vi "rt_main.vi"() -> ()   [LabVIEW 2013]
uses:
  <vilib>/dex/Flush And Wait Empty Condition.ctl
  <vilib>/Platform/TimedLoop/XDataNode/timing_clust.ctl
  <vilib>/Platform/TimedLoop/XDataNode/nitl_modes.ctl
  <vilib>/Platform/TimedLoop/XDataNode/wakeup.ctl
  <vilib>/FPGAPlugInAG/sbRIO-9636/niLvFpga_Open_sbRIO-9636.vi
  <vilib>/rvi/interface/common/dynamic/niFpgaDynamicAddResources.vi
  <vilib>/rvi/interface/common/niFpgaWaitOnOcc.vi
  <vilib>/Utility/error.llb/Error Cluster From Error Code.vi
  <vilib>/rvi/errors/niLvFpgaAdjustHostInterfaceError.vi
  <vilib>/FPGAPlugInAG/Dynamic/niLvFpga_Close_Dynamic.vi
  <vilib>/Platform/TimedLoop/XDataNode/XDataNode.xnode
  <vilib>/rvi/interface/nirviOpenFPGA/nirviOpenFPGA.xnode
  FPGA Bitfiles/ControlPanelproj_FPGATarget_fpgamain_xa8pjD6vMWE.lvbitx
  fpga_main.vi
  <vilib>/rvi/interface/nirviMethod/nirviMethod.xnode
  <vilib>/rvi/interface/nirviReadWriteControl/nirviReadWriteControl.xnode
  <vilib>/rvi/interface/nirviCloseFPGA/nirviCloseFPGA.xnode
  <vilib>/Platform/TimedLoop/XDataNode/XDNodeRunTimeDep.lvlib
  <vilib>/rvi/errors/niLvFpgaMergeErrorWithErrorCode.vi
  <vilib>/FPGAPlugInAG/Dynamic/niLvFpga_ReadFifo_Dynamic.vi
  <vilib>/FPGAPlugInAG/Dynamic/niLvFpga_ConfigureFifo_Dynamic.vi
  NiFpgaLv.dll
  <vilib>/rvi/interface/Simulation/niFpgaSimulationCallBeginRW.vi
  <vilib>/FPGAPlugInAG/Dynamic/niLvFpga_WriteFifo_Dynamic.vi
panel:
  in  "Ignore Minutes and Seconds":bool
  in  "HrStartDispense":i64
  in  "HrGetOrigDispense":i64
  in  "Ignore Minutes and Seconds for ContUpdate":bool
  in  "HrToUpdateCont":i64
  out "Time in 64 Bits":i64
  out "Skip Count":i32
  out "Elements Remaining":u32
  out "Number of Elements":u32
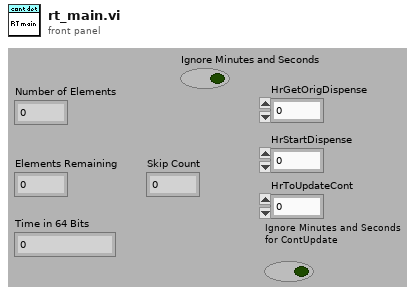
[diagram p1: front panel]
types:
  T1 = typedef "Flush And Wait Empty Condition.ctl" = u8
  T2 = typedef "XDNodeRunTimeDep.lvlib/timing_clust.ctl" = cluster{"Expected End [f-1]":u64, "Actual End [f-1]":u64, "Finished Late? [f-1]":bool, "Expected End [i-1]":u64, "Actual End [i-1]":u64, "Finished Late? [i-1]":bool, "Expected Start [i]":u64, "Actual Start [i]":u64, "Expected Start [f]":u64, "Actual Start [f]":u64, "Source Name":string, "Structure Name":string, "Period":i64, "Deadline":i64, "Offset":i64, "Start":i64, "Priority":i32, "Timeout":i32, "Mode":T3, "Wakeup Reason":T4, "Error":errorcluster, "Source Type":string, "Secondary Source Type":string, "Global End Time":u64, "Global Start Time":u64, "Frame Duration":u64, "Iteration Duration":u64, "Assigned CPU":i32, "I/O Scan Engine Mode":u32}
  T3 = typedef "XDNodeRunTimeDep.lvlib/nitl_modes.ctl" = enum32{"No Change", "Process missed periods, maintain original phase", "Discard missed periods, maintain original phase", "Process missed periods, ignore original phase", "Discard missed periods, ignore original phase"}
  T4 = typedef "XDNodeRunTimeDep.lvlib/wakeup.ctl" = enum32{"Normal", "Aborted", "Asynchronous wakeup", "Timing source error", "Timed loop error", "Timeout"}
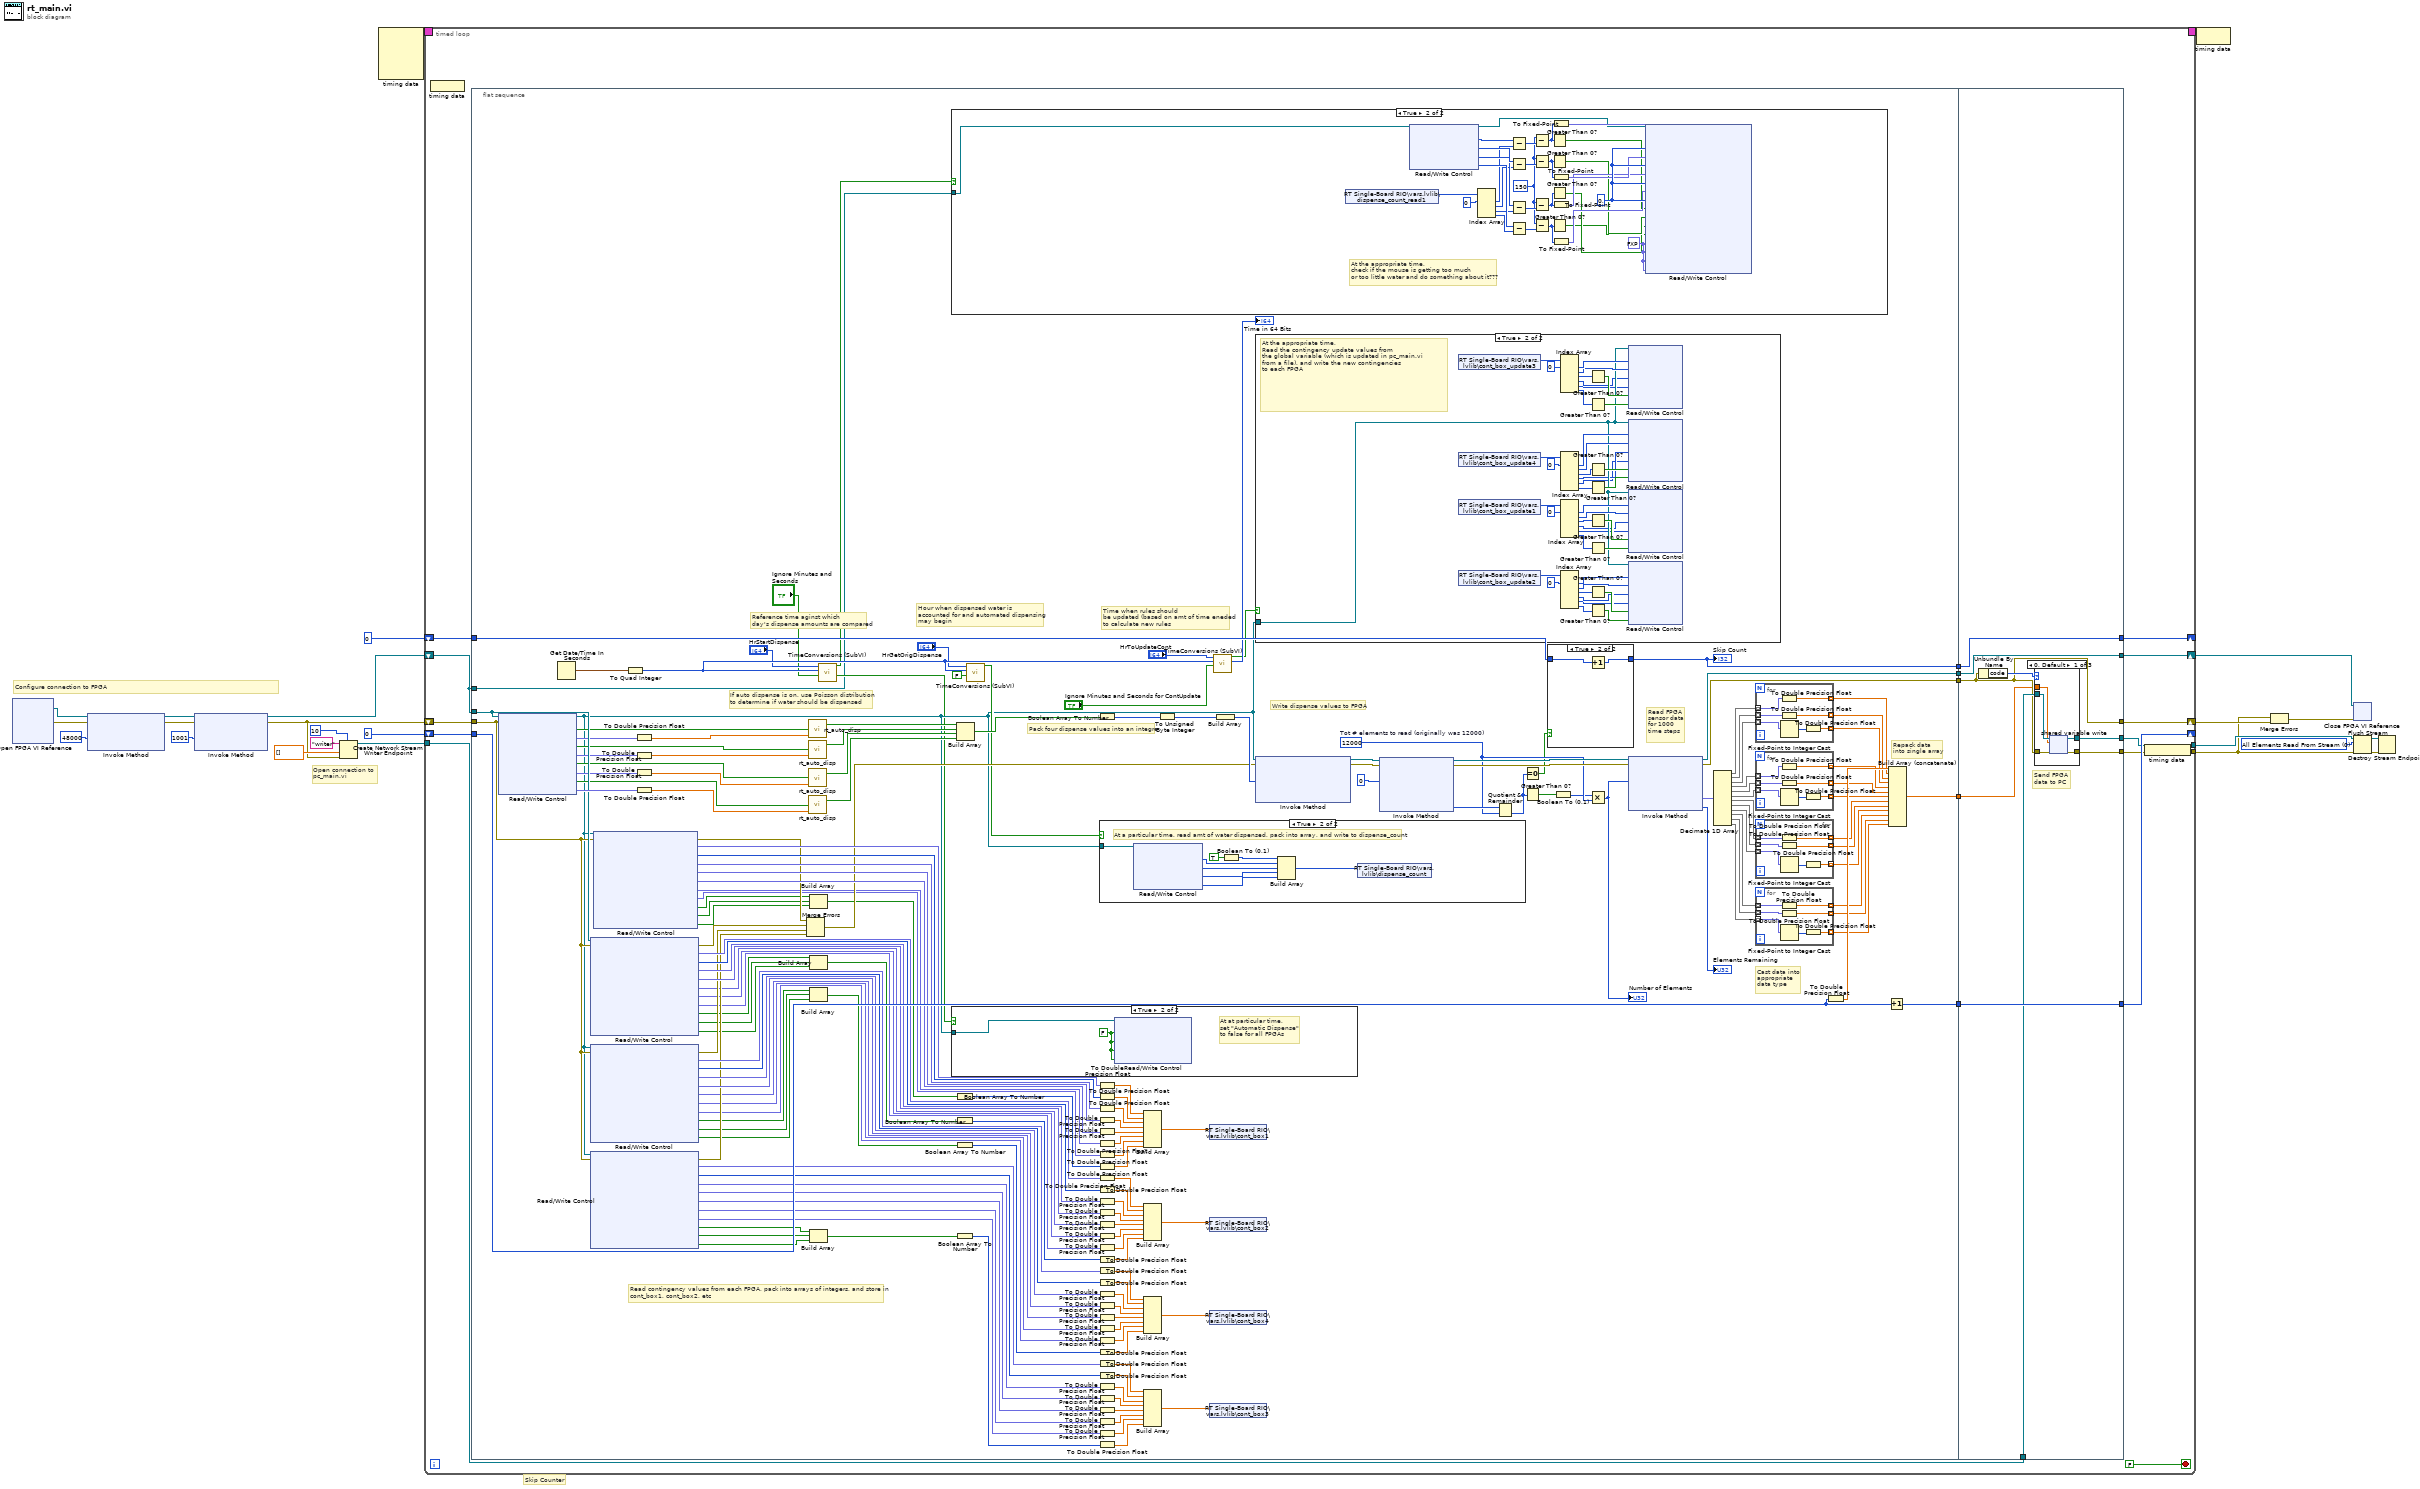
[diagram p0: block diagram]
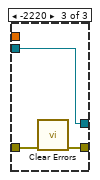
[diagram p8: hidden frame]
diagram:
  w5 = T1 0 items=["All Elements Read From Stream", "All Elements Available for Reading"] ("wait condition")
  # "Open connection to \npc_main.vi"
  # "Configure connection to FPGA"
  # "Skip Counter"
  n1 = xnode "Open FPGA VI Reference"() -> ("FPGA VI Reference Out"=w15:refnum<k20>, "error out"=w14:errorcluster)  [unwired: 2 in]
  n2 = xnode "Invoke Method"("FPGA VI Reference In"=w15, "error in"=w14, "Requested Depth"=u32 48000) -> ("FPGA VI Reference Out"=w9:refnum<k20>, "error out"=w10:errorcluster)  [unwired: 1 out]
  n3 = xnode "Invoke Method"("FPGA VI Reference In"=w9, "error in"=w10, "Requested Depth"=u32 1001) -> ("FPGA VI Reference Out"=w8:refnum<k20>, "error out"=w7:errorcluster)  [unwired: 1 out]
  n4 = Create Network Stream Writer Endpoint(7:10 ("writer buffer size"), 8:w7, 9:dbl[] [], 11:"writer" ("writer name")) -> (3:w6:refnum<k21>)  [unwired: 3 in, 1 out]
  n5 = node-c288() -> (w24:T2)  [unwired: 4 in]
  n6 = timed-loop {
    shift-right: [w41] -> w18
    shift-left: w7 -> [w35]
    timing: w24 -> [_]
    timing-out: [_] -> w23
    shift-right: [w40] -> w22
    shift-left: w8 -> [w25]
    shift-right: [w39] -> _
    shift-left: u32 0 ("index") -> [w38]
    shift-right: [w36] -> _
    shift-left: 0 -> [w37]
    tunnel: w6 -> [w30]
    tunnel: [w29] -> w1
    tunnel: [w28] -> w2
    stop <- FALSE stop-if-true
    n7 = node-c288() -> ()  [unwired: 1 in]
    n8 = flat-sequence {
      tunnel: w38 -> [w205]
      tunnel: w37 -> [w198]
      tunnel: w25 -> [w164]
      tunnel: w35 -> [w120]
      tunnel: [w50] -> w34
      tunnel: [w206] -> w33
      tunnel: [w196] -> w32
      tunnel: [w95] -> w27
      tunnel: [w94] -> w26
      tunnel: w25 -> [w44]
      tunnel: [w333] -> w36
      tunnel: [w334] -> w39
      tunnel: [w335] -> w40
      tunnel: [w328] -> w41
      tunnel: w34 -> [w335]
      tunnel: w33 -> [w334]
      tunnel: w32 -> [w333]
      tunnel: w30 -> [w331]
      tunnel: [w330] -> w29
      tunnel: [w329] -> w28
      tunnel: w27 -> [w328]
      tunnel: w26 -> [w327]
      frame #0 {
        w199 = u32 12000  # Tot # elements to read (originally was 12000)
        # "Reference time aginst which\nday's dispense amounts are compared"
        # "Hour when dispensed water is \naccounted for and automated dispensing\nmay begin"
        # "Time when rules should\nbe updated (based on amt of time eneded\nto calculate new rules"
        # "Read contingency values from each FPGA, pack into arrays of integers, and store in\ncont_box1, cont_box2, etc"
        # "Repack data\ninto single array"
        # "Cast data into\nappropriate\ndata type"
        # "Read FPGA \nsensor data\nfor 1000 \ntime steps"
        # "Write dispense values to FPGA"
        # "Pack four dispense values into an integre"
        # "If auto dispense is on, use Poisson distribution\nto determine if water should be dispensed"
        n9 = xnode "Read/Write Control"("FPGA VI Reference In"=w164, "error in"=w120) -> ("FPGA VI Reference Out"=w49:refnum<k20>, "Automatic Dispense 1"=w111:bool, "Mean 1"=w112:fxp<+,22,9>, "Automatic Dispense 2"=w110:bool, "Mean 2"=w109:fxp<+,22,9>, "Automatic Dispense 3"=w108:bool, "Mean 3"=w107:fxp<+,22,9>, "Automatic Dispense 4"=w113:bool, "Mean 4"=w180:fxp<+,22,9>)  [unwired: 1 out]
        n10 = Get Date/Time In Seconds() -> (seconds since 1Jan1904=w57:timestamp)
        n11 = xnode "Read/Write Control"("FPGA VI Reference In"=w164, "error in"=w120) -> ("error out"=w118:errorcluster, "Outer Threshold 2"=w163:fxp<+,22,9>, "Hold Duration 2"=w161:i16, "Inner Threshold 2"=w159:fxp<+,22,9>, "Min Angle 2"=w156:fxp<+,9,9>, "Max Angle 2"=w60:fxp<+,9,9>, "Min Angle 2 2"=w59:fxp<+,9,9>, "Max Angle 2 2"=w58:fxp<+,9,9>, "Sequence Override 2"=w104:bool, "Override Fail when moved out 2"=w103:bool, "Override Approach 2"=w76:bool)  [unwired: 1 out]
        n12 = xnode "Read/Write Control"("FPGA VI Reference In"=w49, "error in"=w120) -> ("error out"=w119:errorcluster, "Outer Threshold 4"=w132:fxp<+,22,9>, "Hold Duration 4"=w130:i16, "Inner Threshold 4"=w128:fxp<+,22,9>, "Min Angle 4"=w125:fxp<+,9,9>, "Max Angle 4"=w63:fxp<+,9,9>, "Min Angle 4 2"=w62:fxp<+,9,9>, "Max Angle 4 2"=w61:fxp<+,9,9>, "Sequence Override 4"=w96:bool, "Override Fail when moved out 4"=w80:bool, "Override Approach 4"=w79:bool)  [unwired: 1 out]
        n13 = xnode "Read/Write Control"("FPGA VI Reference In"=w49, "error in"=w120) -> ("error out"=w121:errorcluster, "Outer Threshold 3"=w142:fxp<+,22,9>, "Hold Duration 3"=w140:i16, "Inner Threshold 3"=w138:fxp<+,22,9>, "Min Angle 3"=w135:fxp<+,9,9>, "Max Angle 3"=w66:fxp<+,9,9>, "Min Angle 3 2"=w65:fxp<+,9,9>, "Max Angle 3 2"=w64:fxp<+,9,9>, "Sequence Override 3"=w100:bool, "Override Fail when moved out 3"=w99:bool, "Override Approach 3"=w77:bool)  [unwired: 1 out]
        n14 = xnode "Read/Write Control"("FPGA VI Reference In"=w49, "error in"=w120) -> ("error out"=w117:errorcluster, "Outer Threshold 1"=w153:fxp<+,22,9>, "Hold Duration 1"=w151:i16, "Inner Threshold 1"=w149:fxp<+,22,9>, "Min Angle 1"=w146:fxp<+,9,9>, "Max Angle 1"=w145:fxp<+,9,9>, "Min Angle 1 2"=w82:fxp<+,9,9>, "Max Angle 1 2"=w83:fxp<+,9,9>, "Sequence Override 1"=w116:bool, "Override Fail when moved out"=w78:bool, "Override Approach 1"=w81:bool)  [unwired: 1 out]
        n15 = To Quad Integer(1:w57) -> (0:w53:i64)
        n16 = To Double Precision Float(number=w112) -> (double precision float=w179:dbl)
        n17 = To Double Precision Float(number=w109) -> (double precision float=w187:dbl)
        n18 = To Double Precision Float(number=w107) -> (double precision float=w186:dbl)
        n19 = To Double Precision Float(number=w180) -> (double precision float=w181:dbl)
        n20 = Merge Errors(w117, w118, w119, w121) -> (w122:errorcluster)
        n21 = call "rt_auto_disp.vi"("Mean"=w179, "Enable"=w111) -> ("Dispense"=w178:bool)  [unwired: 2 in]
        n22 = call "rt_auto_disp.vi"("Mean"=w187, "Enable"=w110) -> ("Dispense"=w184:bool)  [unwired: 2 in]
        n23 = call "rt_auto_disp.vi"("Mean"=w186, "Enable"=w108) -> ("Dispense"=w185:bool)  [unwired: 2 in]
        n24 = call "rt_auto_disp.vi"("Mean"=w181, "Enable"=w113) -> ("Dispense"=w177:bool)  [unwired: 2 in]
        n25 = Build Array(w116, w78, w81) -> (w115:bool[])
        n26 = Build Array(w104, w103, w76) -> (w106:bool[])
        n27 = Build Array(w96, w80, w79) -> (w98:bool[])
        n28 = Build Array(w100, w99, w77) -> (w102:bool[])
        n29 = call "TimeConversions (SubVI).vi"("Ignore Minutes and Seconds"="Ignore Minutes and Seconds", "Current time"=w53, "HrToUpdate"="HrStartDispense") -> ("Delay_cont"=w47:bool, "Boolean"=w48:bool)  [unwired: 6 in, 1 out]
        n30 = case shown="True" w48 {
          tunnel: w44 -> [_ w219]
          frame False {
          }
          frame True {
            w221 = u16 150 ("x")
            w234 = fxp<+,22,9> 10.0 ("Mean 4")
            w235 = i16 0 ("Automated Pellets Dispensed 2")
            # "At the appropriate time,\ncheck if the mouse is getting too much \nor too little water and do something about it???"
            n31 = shared-variable "RT Single-Board RIO\\vars.lvlib\\dispense_count_read1"() -> (w220:u16[])  [unwired: 1 in, 1 out]
            n32 = xnode "Read/Write Control"("FPGA VI Reference In"=w219) -> ("FPGA VI Reference Out"=w218:refnum<k20>, "Pellets Dispensed 1"=w244:u16, "Pellets Dispensed 2"=w243:u16, "Pellets Dispensed 3"=w242:u16, "Pellets Dispensed 4"=w241:u16)  [unwired: 1 in, 1 out]
            n33 = Index Array(array=w220, index #1=0 ("index")) -> (element #1=w239:u16, element #2=w238:u16, element #3=w237:u16, element #4=w236:u16)  [unwired: 3 in]
            n34 = Subtract(x=w244, y=w239) -> (x-y=w222:u16)
            n35 = Subtract(x=w243, y=w238) -> (x-y=w223:u16)
            n36 = Subtract(x=w242, y=w237) -> (x-y=w224:u16)
            n37 = Subtract(x=w241, y=w236) -> (x-y=w225:u16)
            n38 = Subtract(x=w221, y=w222) -> (x-y=w214:i16)
            n39 = Subtract(x=w221, y=w223) -> (x-y=w215:i16)
            n40 = Subtract(x=w221, y=w224) -> (x-y=w217:i16)
            n41 = Subtract(x=w221, y=w225) -> (x-y=w216:i16)
            n42 = Greater Than 0?(x=w214) -> (x > 0?=w229:bool)
            n43 = Greater Than 0?(x=w215) -> (x > 0?=w228:bool)
            n44 = Greater Than 0?(x=w217) -> (x > 0?=w227:bool)
            n45 = Greater Than 0?(x=w216) -> (x > 0?=w226:bool)
            n46 = To Fixed-Point(number=w214) -> (fixed-point=w233:fxp<+,10,10>)  [unwired: 1 in]
            n47 = To Fixed-Point(number=w215) -> (fixed-point=w232:fxp<+,10,10>)  [unwired: 1 in]
            n48 = To Fixed-Point(number=w217) -> (fixed-point=w231:fxp<+,10,10>)  [unwired: 1 in]
            n49 = To Fixed-Point(number=w216) -> (fixed-point=w230:fxp<+,10,10>)  [unwired: 1 in]
            n50 = xnode "Read/Write Control"("FPGA VI Reference In"=w218, "Automated Pellets Target 1"=w233, "Automated Pellets Dispensed 1"=w235, "Automated Pellets Target 2"=w232, "Automated Pellets Dispensed 2"=w235, "Automated Pellets Target 3"=w231, "Automated Pellets Dispensed 3"=w235, "Automated Pellets Target 4"=w230, "Automated Pellets Dispensed 4"=w235, "Automatic Dispense 1"=w229, "Automatic Dispense 2"=w228, "Automatic Dispense 3"=w227, "Automatic Dispense 4"=w226, "Mean 1"=w234, "Mean 2"=w234, "Mean 3"=w234, "Mean 4"=w234) -> ()  [unwired: 1 in, 2 out]
          }
        }
        n51 = case shown="True" w47 {
          tunnel: w49 -> [_ w253]
          frame False {
          }
          frame True {
            w254 = FALSE ("Automatic Dispense 1")
            # "At at particular time,\nset \"Automatic Dispense\"\nto false for all FPGAs"
            n52 = xnode "Read/Write Control"("FPGA VI Reference In"=w253, "Automatic Dispense 1"=w254, "Automatic Dispense 2"=w254, "Automatic Dispense 3"=w254, "Automatic Dispense 4"=w254) -> ()  [unwired: 1 in, 2 out]
          }
        }
        n53 = Boolean Array To Number(Boolean array=w115) -> (number=w114:u32)
        n54 = Boolean Array To Number(Boolean array=w106) -> (number=w105:u32)
        n55 = Boolean Array To Number(Boolean array=w98) -> (number=w97:u32)
        n56 = Boolean Array To Number(Boolean array=w102) -> (number=w101:u32)
        n57 = Build Array(w178, w184, w185, w177) -> (w188:bool[])
        n58 = call "TimeConversions (SubVI).vi"("Ignore Minutes and Seconds"=FALSE, "Current time"=w53, "HrToUpdate"="HrGetOrigDispense") -> ("Boolean"=w51:bool)  [unwired: 6 in, 2 out]
        n59 = Boolean Array To Number(Boolean array=w188) -> (number=w189:u32)
        n60 = To Double Precision Float(number=w153) -> (double precision float=w152:dbl)
        n61 = To Double Precision Float(number=w151) -> (double precision float=w150:dbl)
        n62 = To Double Precision Float(number=w149) -> (double precision float=w148:dbl)
        n63 = To Double Precision Float(number=w146) -> (double precision float=w147:dbl)
        n64 = To Double Precision Float(number=w145) -> (double precision float=w144:dbl)
        n65 = To Double Precision Float(number=w82) -> (double precision float=w84:dbl)
        n66 = To Double Precision Float(number=w83) -> (double precision float=w85:dbl)
        n67 = To Double Precision Float(number=w114) -> (double precision float=w86:dbl)
        n68 = To Double Precision Float(number=w163) -> (double precision float=w162:dbl)
        n69 = To Double Precision Float(number=w161) -> (double precision float=w160:dbl)
        n70 = To Double Precision Float(number=w159) -> (double precision float=w158:dbl)
        n71 = To Double Precision Float(number=w156) -> (double precision float=w157:dbl)
        n72 = To Double Precision Float(number=w60) -> (double precision float=w155:dbl)
        n73 = To Double Precision Float(number=w59) -> (double precision float=w73:dbl)
        n74 = To Double Precision Float(number=w58) -> (double precision float=w74:dbl)
        n75 = To Double Precision Float(number=w105) -> (double precision float=w75:dbl)
        n76 = To Double Precision Float(number=w132) -> (double precision float=w131:dbl)
        n77 = To Double Precision Float(number=w130) -> (double precision float=w129:dbl)
        n78 = To Double Precision Float(number=w128) -> (double precision float=w127:dbl)
        n79 = To Double Precision Float(number=w125) -> (double precision float=w126:dbl)
        n80 = To Double Precision Float(number=w63) -> (double precision float=w124:dbl)
        n81 = To Double Precision Float(number=w62) -> (double precision float=w71:dbl)
        n82 = To Double Precision Float(number=w61) -> (double precision float=w70:dbl)
        n83 = To Double Precision Float(number=w97) -> (double precision float=w72:dbl)
        n84 = To Double Precision Float(number=w142) -> (double precision float=w141:dbl)
        n85 = To Double Precision Float(number=w140) -> (double precision float=w139:dbl)
        n86 = To Double Precision Float(number=w138) -> (double precision float=w137:dbl)
        n87 = To Double Precision Float(number=w135) -> (double precision float=w136:dbl)
        n88 = To Double Precision Float(number=w66) -> (double precision float=w134:dbl)
        n89 = To Double Precision Float(number=w65) -> (double precision float=w67:dbl)
        n90 = To Double Precision Float(number=w64) -> (double precision float=w68:dbl)
        n91 = To Double Precision Float(number=w101) -> (double precision float=w69:dbl)
        n92 = case shown="True" w51 {
          tunnel: w49 -> [_ w252]
          frame False {
          }
          frame True {
            # "At a particular time, read amt of water dispensed, pack into array, and write to dispense_count"
            n93 = xnode "Read/Write Control"("FPGA VI Reference In"=w252) -> ("Pellets Dispensed 1"=w248:u16, "Pellets Dispensed 2"=w249:u16, "Pellets Dispensed 3"=w250:u16, "Pellets Dispensed 4"=w251:u16)  [unwired: 1 in, 2 out]
            n94 = Boolean To (0,1)(Boolean=TRUE) -> (0, 1=w246:i16)
            n95 = Build Array(w246, w248, w249, w250, w251) -> (w245:u16[])
            n96 = shared-variable "RT Single-Board RIO\\vars.lvlib\\dispense_count"(w245) -> ()  [unwired: 1 in, 1 out]
          }
        }
        n97 = Build Array(w152, w150, w148, w147, w144, w84, w85, w86) -> (w143:dbl[])
        n98 = Build Array(w162, w160, w158, w157, w155, w73, w74, w75) -> (w154:dbl[])
        n99 = Build Array(w131, w129, w127, w126, w124, w71, w70, w72) -> (w123:dbl[])
        n100 = Build Array(w141, w139, w137, w136, w134, w67, w68, w69) -> (w133:dbl[])
        n101 = To Unsigned Byte Integer(number=w189) -> (unsigned 8bit integer=w183:u8)
        n102 = shared-variable "RT Single-Board RIO\\vars.lvlib\\cont_box1"(w143) -> ()  [unwired: 1 in, 1 out]
        n103 = shared-variable "RT Single-Board RIO\\vars.lvlib\\cont_box2"(w154) -> ()  [unwired: 1 in, 1 out]
        n104 = shared-variable "RT Single-Board RIO\\vars.lvlib\\cont_box4"(w123) -> ()  [unwired: 1 in, 1 out]
        n105 = shared-variable "RT Single-Board RIO\\vars.lvlib\\cont_box3"(w133) -> ()  [unwired: 1 in, 1 out]
        n106 = call "TimeConversions (SubVI).vi"("Ignore Minutes and Seconds"="Ignore Minutes and Seconds for ContUpdate", "Current time"=w53, "HrToUpdate"="HrToUpdateCont") -> ("Time in 64 Bits"=→"Time in 64 Bits":i64, "Boolean"=w46:bool)  [unwired: 6 in, 1 out]
        n107 = Build Array(w183) -> (w182:u8[])
        n108 = case shown="True" w46 {
          tunnel: w49 -> [_ w271]
          frame False {
          }
          frame True {
            # "At the appropriate time,\nRead the contingency update values from\nthe global variable (which is updated in pc_main.vi\nfrom a file), and write the new contingencies\nto each FPGA"
            n109 = shared-variable "RT Single-Board RIO\\vars.lvlib\\cont_box_update3"() -> (w273:i32[])  [unwired: 1 in, 1 out]
            n110 = shared-variable "RT Single-Board RIO\\vars.lvlib\\cont_box_update4"() -> (w272:i32[])  [unwired: 1 in, 1 out]
            n111 = shared-variable "RT Single-Board RIO\\vars.lvlib\\cont_box_update1"() -> (w275:i32[])  [unwired: 1 in, 1 out]
            n112 = shared-variable "RT Single-Board RIO\\vars.lvlib\\cont_box_update2"() -> (w274:i32[])  [unwired: 1 in, 1 out]
            n113 = Index Array(array=w273, index #1=0 ("index")) -> (element #1=w279:i32, element #2=w278:i32, element #3=w262:i32, element #4=w260:i32, element #5=w259:i32, element #6=w261:i32)  [unwired: 5 in]
            n114 = Index Array(array=w272, index #1=0 ("index")) -> (element #1=w281:i32, element #2=w280:i32, element #3=w270:i32, element #4=w269:i32, element #5=w268:i32, element #6=w267:i32)  [unwired: 5 in]
            n115 = Index Array(array=w275, index #1=0 ("index")) -> (element #1=w283:i32, element #2=w282:i32, element #3=w266:i32, element #4=w264:i32, element #5=w263:i32, element #6=w265:i32)  [unwired: 5 in]
            n116 = Index Array(array=w274, index #1=0 ("index")) -> (element #1=w276:i32, element #2=w277:i32, element #3=w258:i32, element #4=w256:i32, element #5=w255:i32, element #6=w257:i32)  [unwired: 5 in]
            n117 = Greater Than 0?(x=w262) -> (x > 0?=w292:bool)
            n118 = Greater Than 0?(x=w261) -> (x > 0?=w293:bool)
            n119 = Greater Than 0?(x=w270) -> (x > 0?=w295:bool)
            n120 = Greater Than 0?(x=w267) -> (x > 0?=w294:bool)
            n121 = Greater Than 0?(x=w266) -> (x > 0?=w289:bool)
            n122 = Greater Than 0?(x=w265) -> (x > 0?=w288:bool)
            n123 = Greater Than 0?(x=w258) -> (x > 0?=w291:bool)
            n124 = Greater Than 0?(x=w257) -> (x > 0?=w290:bool)
            n125 = xnode "Read/Write Control"("FPGA VI Reference In"=w271, "Min Angle 3"=w279, "Max Angle 3"=w278, "Min Angle 3 2"=w260, "Max Angle 3 2"=w259, "CCW(T)  3"=w292, "CCW(T)  3 2"=w293) -> ()  [unwired: 1 in, 2 out]
            n126 = xnode "Read/Write Control"("FPGA VI Reference In"=w271, "Min Angle 4"=w281, "Max Angle 4"=w280, "Min Angle 4 2"=w269, "Max Angle 4 2"=w268, "CCW(T)  4"=w295, "CCW(T)  4 2"=w294) -> ()  [unwired: 1 in, 2 out]
            n127 = xnode "Read/Write Control"("FPGA VI Reference In"=w271, "Min Angle 1"=w283, "Max Angle 1"=w282, "Min Angle 1 2"=w264, "Max Angle 1 2"=w263, "CCW(T) 1"=w289, "CCW(T) 1 2"=w288) -> ()  [unwired: 1 in, 2 out]
            n128 = xnode "Read/Write Control"("FPGA VI Reference In"=w271, "Min Angle 2"=w276, "Max Angle 2"=w277, "Min Angle 2 2"=w256, "Max Angle 2 2"=w255, "CCW(T)  2"=w291, "CCW(T)  2 2"=w290) -> ()  [unwired: 1 in, 2 out]
          }
        }
        n129 = xnode "Invoke Method"("FPGA VI Reference In"=w49, "error in"=w122, "Data"=w182) -> ("FPGA VI Reference Out"=w208:refnum<k20>, "error out"=w207:errorcluster)  [unwired: 1 in, 1 out]
        n130 = xnode "Invoke Method"("FPGA VI Reference In"=w208, "error in"=w207, "Number of Elements"=u32 0) -> ("FPGA VI Reference Out"=w211:refnum<k20>, "error out"=w210:errorcluster, "Elements Remaining"=w212:u32)  [unwired: 1 in, 1 out]
        n131 = Quotient & Remainder(x=w212, y=w199) -> (floor(x/y)=w93:u32)  [unwired: 1 out]
        n132 = Equal To 0?(x=w93) -> (x = 0?=w197:bool)
        n133 = Greater Than 0?(x=w93) -> (x > 0?=w91:bool)
        n134 = case shown="True" w197 {
          tunnel: w198 -> [w310 w312]
          tunnel: [w310 w311] -> w196
          frame False {
          }
          frame True {
            n135 = Increment(x=w312) -> (x+1=w311:i32)
          }
        }
        "Skip Count" <- w196
        n136 = Boolean To (0,1)(Boolean=w91) -> (0, 1=w92:i16)
        n137 = Multiply(x=w92, y=w199) -> (x*y=w204:u32)
        "Number of Elements" <- w204
        n138 = xnode "Invoke Method"("FPGA VI Reference In"=w211, "error in"=w210, "Number of Elements"=w204) -> ("FPGA VI Reference Out"=w50:refnum<k20>, "error out"=w95:errorcluster, "Data"=w209:fxp<+/-,22,10>[], "Elements Remaining"=→"Elements Remaining":u32)  [unwired: 1 in]
        n139 = Decimate 1D Array(w209) -> (w89:fxp<+/-,22,10>[], w88:fxp<+/-,22,10>[], w87:fxp<+/-,22,10>[], w203:fxp<+/-,22,10>[], w202:fxp<+/-,22,10>[], w201:fxp<+/-,22,10>[], w176:fxp<+/-,22,10>[], w175:fxp<+/-,22,10>[], w174:fxp<+/-,22,10>[], w173:fxp<+/-,22,10>[], w172:fxp<+/-,22,10>[], w171:fxp<+/-,22,10>[])
        n140 = for {
          tunnel: w89 -> [w326] mode=indexing
          tunnel: w88 -> [w325] mode=indexing
          tunnel: w87 -> [w324] mode=indexing
          tunnel: [w321] -> w195 mode=indexing
          tunnel: [w320] -> w194 mode=indexing
          tunnel: [w322] -> w193 mode=indexing
          n141 = To Double Precision Float(number=w326) -> (double precision float=w321:dbl)
          n142 = To Double Precision Float(number=w325) -> (double precision float=w320:dbl)
          n143 = Fixed-Point to Integer Cast(1:w324) -> (0:w323:i32)
          n144 = To Double Precision Float(number=w323) -> (double precision float=w322:dbl)
        }
        n145 = for {
          tunnel: w203 -> [w319] mode=indexing
          tunnel: w202 -> [w318] mode=indexing
          tunnel: w201 -> [w317] mode=indexing
          tunnel: [w314] -> w192 mode=indexing
          tunnel: [w313] -> w191 mode=indexing
          tunnel: [w315] -> w190 mode=indexing
          n146 = To Double Precision Float(number=w319) -> (double precision float=w314:dbl)
          n147 = To Double Precision Float(number=w318) -> (double precision float=w313:dbl)
          n148 = Fixed-Point to Integer Cast(1:w317) -> (0:w316:i32)
          n149 = To Double Precision Float(number=w316) -> (double precision float=w315:dbl)
        }
        n150 = for {
          tunnel: w176 -> [w309] mode=indexing
          tunnel: w175 -> [w308] mode=indexing
          tunnel: w174 -> [w307] mode=indexing
          tunnel: [w304] -> w170 mode=indexing
          tunnel: [w303] -> w169 mode=indexing
          tunnel: [w305] -> w168 mode=indexing
          n151 = To Double Precision Float(number=w309) -> (double precision float=w304:dbl)
          n152 = To Double Precision Float(number=w308) -> (double precision float=w303:dbl)
          n153 = Fixed-Point to Integer Cast(1:w307) -> (0:w306:i32)
          n154 = To Double Precision Float(number=w306) -> (double precision float=w305:dbl)
        }
        n155 = for {
          tunnel: w173 -> [w302] mode=indexing
          tunnel: w171 -> [w301] mode=indexing
          tunnel: [w298] -> w167 mode=indexing
          tunnel: [w297] -> w166 mode=indexing
          tunnel: [w299] -> w165 mode=indexing
          tunnel: w172 -> [w296] mode=indexing
          n156 = To Double Precision Float(number=w302) -> (double precision float=w298:dbl)
          n157 = To Double Precision Float(number=w296) -> (double precision float=w297:dbl)
          n158 = Fixed-Point to Integer Cast(1:w301) -> (0:w300:i32)
          n159 = To Double Precision Float(number=w300) -> (double precision float=w299:dbl)
        }
        n160 = To Double Precision Float(number=w205) -> (double precision float=w200:dbl)
        n161 = Increment(x=w205) -> (x+1=w206:u32)
        n162 = Build Array (concatenate)(w200, w195, w194, w193, w192, w191, w190, w170, w169, w168, w167, w166, w165) -> (w94:dbl[])
      }
      frame #1 {
        # "Send FPGA \ndata to PC"
        n163 = Unbundle By Name(w328) -> ("code"=w332:i32)
        n164 = case shown="0, Default" w332 {
          tunnel: w328 -> [w336 w342 w345]
          tunnel: [w339 w342 w344] -> w330
          tunnel: w331 -> [w338 w341 w343]
          tunnel: [w340 w341 w343] -> w329
          tunnel: w327 -> [w337 _ _]
          frame 0, Default {
            n165 = shared-variable-write(w338, w336, w337) -> (w340:refnum<k21>, w339:errorcluster)  [unwired: 1 in, 1 out]
          }
          frame 2 {
          }
          frame -2220 {
            n166 = call <vilib>:"Clear Errors.vi"("error in (no error)"=w345) -> ("error out"=w344:errorcluster)  [unwired: 6 in]
          }
        }
      }
    }
    n167 = node-c288() -> ()  [unwired: 1 out]
  }
  n168 = node-c288(w23) -> ()
  n169 = Merge Errors(w1, w18) -> (w17:errorcluster)
  n170 = xnode "Close FPGA VI Reference"("FPGA VI Reference In"=w22, "error in"=w17) -> ()  [unwired: 1 out]
  n171 = Flush Stream(8:w1, 10:w5, 11:w2) -> (0:w4:errorcluster, 3:w3:refnum<k21>)  [unwired: 1 in, 1 out]
  n172 = Destroy Stream Endpoint(8:w4, 11:w3) -> ()  [unwired: 1 out]
